vi "enable.vi"(8 "error in (no error)":errorcluster, 11 "DL090603DAQmxOnOffEmissionSensor in":refnum<class "DetectorDL090603DAQmxOnOff.lvclass">=refnum) -> (0 "error out":errorcluster, 3 "DL090603DAQmxOnOffEmissionSensor out":refnum<class "DetectorDL090603DAQmxOnOff.lvclass">)   [LabVIEW 2010, in "DetectorDL090603DAQmxOnOff.lvclass"]
uses:
  DetectorDL090603DAQmxOnOff.lvclass
  DetectorDL090603DAQmxOnOff.lvclass/DetectorDL090603DAQmxOnOff.ctl
  DigitalOut/DigitalOutDL110325DAQmx/DigitalOutDL110325DAQmx/DigitalOutDL110325DAQmx.lvclass
  GenericDetector/GenericDetector/GenericDetector.lvclass
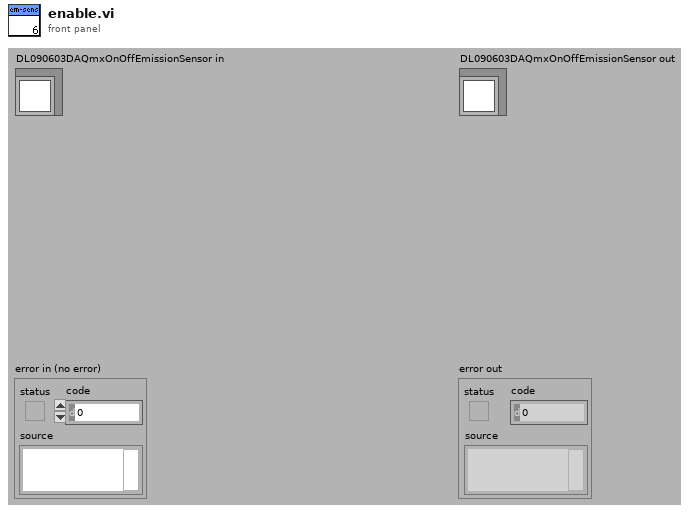
[diagram p1: front panel]
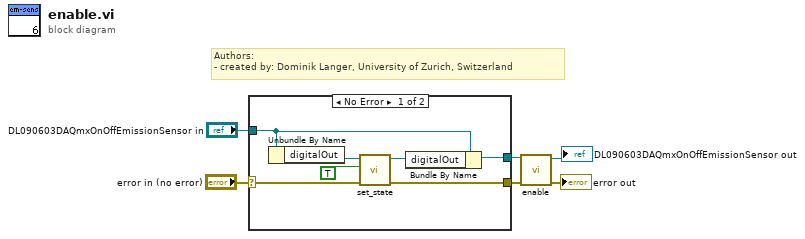
[diagram p0: block diagram]
diagram:
  # "Authors: \n- created by: Dominik Langer, University of Zurich, Switzerland"
  n1 = case shown="No Error" "error in (no error)" {
    selector: "error in (no error)" -> [w11 w15]
    tunnel: [w10 w15] -> w4
    tunnel: [w12 w14] -> w2
    tunnel: "DL090603DAQmxOnOffEmissionSensor in" -> [w13 w14]
    frame No Error {
      n2 = Unbundle By Name(w13) -> ("digitalOut"=w8:refnum<class "DigitalOutDL110325DAQmx.lvclass">)
      n3 = call-dynamic "set_state.vi"("error in (no error)"=w11, "state"=TRUE ("data"), "DAQmxDigitalOut in"=w8) -> ("error out"=w10:errorcluster, "DAQmxDigitalOut out"=w7:refnum<class "DigitalOutDL110325DAQmx.lvclass">)  [unwired: 7 in]
      n4 = Bundle By Name(cluster=w13, "digitalOut"=w7) -> (w12:refnum<class "DetectorDL090603DAQmxOnOff.lvclass">)
    }
    frame Error {
    }
  }
  n5 = call-parent "enable.vi"("error in (no error)"=w4, "GenericEmissionSensor in"=w2) -> ("error out"=→"error out":errorcluster, "GenericEmissionSensor out"=→"DL090603DAQmxOnOffEmissionSensor out":refnum<class "DetectorDL090603DAQmxOnOff.lvclass">)  [unwired: 8 out]
